vi "evaluate_SP_bypass_valve.vi"(7 "PID Range":cluster{"output high":dbl, "output low":dbl}={"output high"=10.0, "output low"=-10.0} {"output low" format="%.2f"; "output high" format="%.2f"}, 8 "ref_sp_ch1":refnum<vi>, 9 "control_step":dbl=0.2 format="%#_13g", 10 "F_org":dbl, 11 "control":dbl) -> (0 "status":u32(colorbox), 3 "F_new":dbl)   [LabVIEW 2019]
panel:
  out "lo":dbl=22.0
  out "hi":dbl=38.0
  in  "range_warn":dbl=0.99
  # "L/m"
  # "L/m"
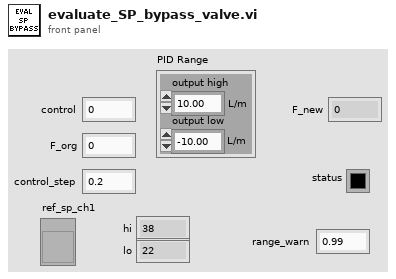
[diagram p1: front panel]
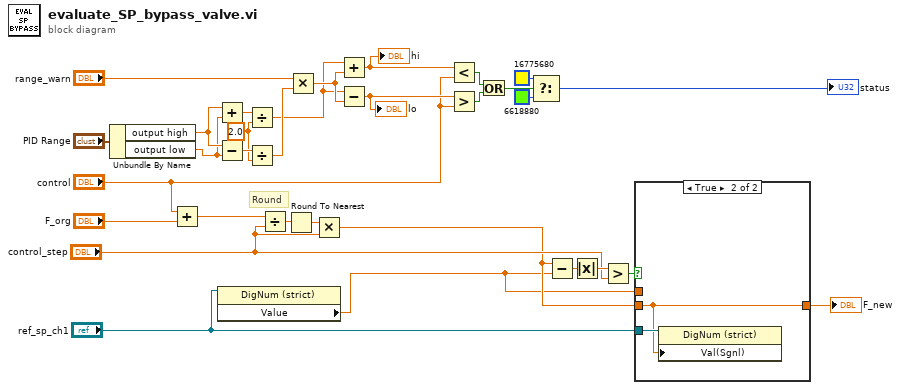
[diagram p0: block diagram]
diagram:
  w16 = 2.0 ("y")
  # "Round"
  n1 = Unbundle By Name("PID Range") -> ("output high"=w11:dbl, "output low"=w10:dbl)
  n2 = Add(x="control", y="F_org") -> (x+y=w24:dbl)
  n3 = Add(x=w11, y=w10) -> (x+y=w18:dbl)
  n4 = Subtract(x=w11, y=w10) -> (x-y=w17:dbl)
  n5 = property class="DigNum (strict)"(reference="ref_sp_ch1") -> ("Value"=w3:dbl)  [unwired: 1 in, 2 out]
  n6 = Divide(x=w18, y=w16) -> (x/y=w7:dbl)
  n7 = Divide(x=w17, y=w16) -> (x/y=w8:dbl)
  n8 = Divide(x=w24, y="control_step") -> (x/y=w27:dbl)
  n9 = Round To Nearest(number=w27) -> (nearest integer value=w26:dbl)
  n10 = Multiply(x="range_warn", y=w8) -> (x*y=w15:dbl)
  n11 = Multiply(x=w26, y="control_step") -> (x*y=w6:dbl)
  n12 = Add(x=w7, y=w15) -> (x+y=w14:dbl)
  "hi" <- w14
  n13 = Subtract(x=w7, y=w15) -> (x-y=w13:dbl)
  "lo" <- w13
  n14 = Less?(x=w14, y="control") -> (x < y?=w20:bool)
  n15 = Greater?(x=w13, y="control") -> (0:w21:bool)
  n16 = Or(x=w20, y=w21) -> (x .or. y?=w19:bool)
  n17 = Select(t=u32 16775680 ("alarm_status"), s=w19, f=u32 6618880 ("alarm_status")) -> (s? t:f=→"status":u32)
  n18 = Subtract(x=w6, y=w3) -> (x-y=w31:dbl)
  n19 = Absolute Value(x=w31) -> (abs(x)=w30:dbl)
  n20 = Greater?(x=w30, y="control_step") -> (0:w29:bool)
  n21 = case shown="True" w29 {
    tunnel: "ref_sp_ch1" -> [_ w34]
    tunnel: w6 -> [_ w33]
    tunnel: [w32 w33] -> w4
    tunnel: w3 -> [w32 _]
    frame False {
    }
    frame True {
      n22 = property class="DigNum (strict)"(reference=w34, "Val(Sgnl)"=w33) -> ()  [unwired: 1 in, 2 out]
    }
  }
  "F_new" <- w4
